vi "Teleop.vi"(10 "Match Info":T1={"Autonomous Elapsed Seconds"=0.0, "TeleOp Elapsed Seconds"=0.0, "Disabled Elapsed Seconds"=0.0, "Visited Autonomous"=FALSE, "Visited TeleOp"=FALSE, "Visited Disabled"=FALSE, "Autonomous Settings"={"Autonomous Style"=enum."Independent", "VI Refnum"=refnum}}, 11 "Call Context":T2) -> ()   [LabVIEW 2011]
doc: "This VI is called for each TeleOp packet received from the DS where the robot is not disabled. It is often used to read from the joysticks and update I/O or to update setpoints for timed control loops. It should complete and return within 20 milliseconds or it may miss DS packets."
uses:
  <vilib>/Rock Robotics/WPI/DriverStation/WPI_DriverStationDerivedRobotMode.ctl
  <vilib>/Rock Robotics/WPI/DriverStation/WPI_DriverStationMatch Info.ctl
  <vilib>/Rock Robotics/WPI/Relay/WPI_RelayValue.ctl
  Robot Global Data.vi
  <vilib>/Rock Robotics/WPI/RobotDrive/WPI_RobotDriveArcadeDrive_Standard(NoSaturation).vi
  <vilib>/Rock Robotics/WPI/Compressor/WPI_CompressorGetSetRefNum.vi
panel:
  in  "Time (msec)":u32=500
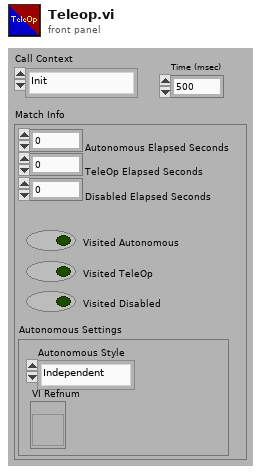
[diagram p1: front panel]
types:
  T1 = typedef "WPI_DriverStationMatch Info.ctl" = cluster{"Autonomous Elapsed Seconds":dbl, "TeleOp Elapsed Seconds":dbl, "Disabled Elapsed Seconds":dbl, "Visited Autonomous":bool, "Visited TeleOp":bool, "Visited Disabled":bool, "Autonomous Settings":cluster{"Autonomous Style":enum16{"Iterative", "Independent"}, "VI Refnum":refnum<vi>}}
  T2 = typedef "WPI_DriverStationDerivedRobotMode.ctl" = enum16{"Init", "Execute", "Stop"}
  T3 = typedef "WPI_RobotDriveDevRef.ctl" = cluster{"DevStatus":errorcluster, "Motors[]":T4[], "Square Inputs":bool, "Max Output":dbl, "Isochronous":bool}
  T4 = typedef "WPI_MotorControlDeviceRef.ctl" = cluster{"DeviceStatus":errorcluster, "Type":enum16{"PWM", "CAN"}, "PWM":cluster{"Digital Module":T5, "PWM Channel":T6, "DeadBand":T7}, "CAN":cluster{"Device Number":u8, "Control Mode":T8, "Semaphore":T9, "Max Vout":dbl}, "Invert":bool, "TransformRef":T10, "InvTransformRef":T10}
  T5 = typedef "FPGA_TypedefDigitalModule.ctl" = enum16{"Digital Module 1", "Digital Module 2"}
  T6 = typedef "FPGA_DIOPWMChannel.ctl" = enum8{"PWM 1", "PWM 2", "PWM 3", "PWM 4", "PWM 5", "PWM 6", "PWM 7", "PWM 8", "PWM 9", "PWM 10", "Invalid"}
  T7 = typedef "WPI_PWMDeadband.ctl" = cluster{"Name":string, "maxPositivePwm":i32, "minPositivePwm":i32, "centerPwm":i32, "maxNegativePwm":i32, "minNegativePwm":i32, "angularRange":u16}
  T8 = typedef "WPI_CANJaguar_ControlMode.ctl" = enum8{"Percent VBus", "Current", "Speed", "Position", "Voltage"}
  T9 = typedef "Semaphore RefNum" = refnum<k1>
  T10 = typedef "WPI_PWMTransform_ConPane.ctl" = refnum<vi>
  T11 = typedef "WPI_JoystickDevRef.ctl" = cluster{"Device":T12}
  T12 = typedef "WPI_JoystickDeviceEnum.ctl" = enum16{"USB 1", "USB 2", "USB 3", "USB 4", "Kinect 1", "Kinect 2"}
  T13 = typedef "WPI_JoystickButtonState.ctl" = cluster{"Button 1":bool, "Button 2":bool, "Button 3":bool, "Button 4":bool, "Button 5":bool, "Button 6":bool, "Button 7":bool, "Button 8":bool, "Button 9":bool, "Button 10":bool, "Button 11":bool, "Button 12":bool}
  T14 = cluster{"axis 1 (x)":dbl, "axis 2 (y)":dbl, "axis 3 (throttle)":dbl, "axis 4":dbl, "axis 5":dbl, "axis 6":dbl}
  T15 = typedef "WPI_RelayDevRef.ctl" = cluster{"DevStatus":errorcluster, "Relay Channel":T16, "Digital Module":T5, "Relay Direction":T17}
  T16 = typedef "FPGA_DIORelayChannel.ctl" = enum8{"Relay 1", "Relay 2", "Relay 3", "Relay 4", "Relay 5", "Relay 6", "Relay 7", "Relay 8", "Invalid"}
  T17 = typedef "WPI_RelayDirection.ctl" = enum16{"Both directions", "Forward only", "Reverse only"}
  T18 = typedef "WPI_CompressorDevRef.ctl" = cluster{"DevStatus":errorcluster, "DigitalInputDevRef":T19, "RelayDevRef":T15}
  T19 = typedef "WPI_DigitalInputDevRef.ctl" = cluster{"DevStatus":errorcluster, "DIO Channel":T20, "Digital Module":T5}
  T20 = typedef "FPGA_DIOChannel.ctl" = enum8{"DIO 1", "DIO 2", "DIO 3", "DIO 4", "DIO 5", "DIO 6", "DIO 7", "DIO 8", "DIO 9", "DIO 10", "DIO 11", "DIO 12", "DIO 13", "DIO 14", "Invalid"}
  T21 = typedef "WPI_RelayValue.ctl" = enum16{"Off", "On", "Forward", "Reverse"}
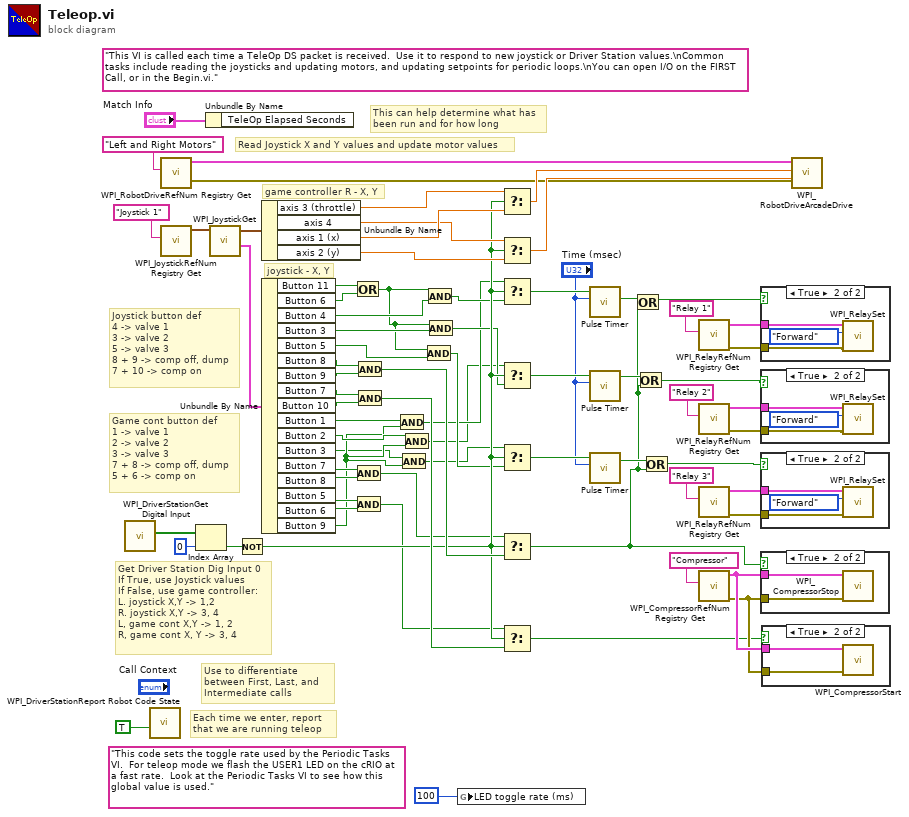
[diagram p0: block diagram]
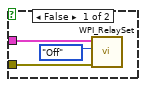
[diagram p2: hidden frame]
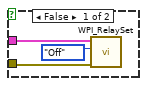
[diagram p3: hidden frame]
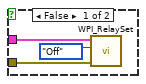
[diagram p4: hidden frame]
diagram:
  (unwired) "This code sets the toggle rate used by the Periodic Tasks VI.  For teleop mode we flash the USER1 LED on the cRIO at a fast rate.  Look at the Periodic Tasks VI to see how this global value is used."
  (unwired) "This VI is called each time a TeleOp DS packet is received.  Use it to respond to new joystick or Driver Station values.\nCommon tasks include reading the joysticks and updating motors, and updating setpoints for periodic loops.\nYou can open I/O on the FIRST Call, or in the Begin.vi."
  # "Joystick button def\n4 -> valve 1\n3 -> valve 2\n5 -> valve 3\n8 + 9 -> comp off, dump\n7 + 10 -> comp on"
  # "joystick - X, Y"
  # "game controller R - X, Y"
  # "Game cont button def\n1 -> valve 1\n2 -> valve 2\n3 -> valve 3\n7 + 8 -> comp off, dump\n5 + 6 -> comp on"
  # "Get Driver Station Dig Input 0\nIf True, use Joystick values\nIf False, use game controller:\nL. joystick X,Y -> 1,2\nR. joystick X,Y -> 3, 4\nL, game cont X,Y -> 1, 2\nR, game cont X, Y -> 3, 4"
  # "Each time we enter, report that we are running teleop"
  # "Use to differentiate between First, Last, and Intermediate calls"
  # "This can help determine what has\nbeen run and for how long"
  # "Read Joystick X and Y values and update motor values"
  n1 = call <vilib>:"WPI_DriverStationGet Digital Input.vi"() -> ("Driver Station Digital Input (1-8)"=w60:bool[])  [unwired: 11 in]
  n2 = call <vilib>:"WPI_DriverStationReport Robot Code State.vi"("TeleOp"=TRUE ("Autonomous")) -> ()  [unwired: 10 in, 1 out]
  n3 = call <vilib>:"WPI_RobotDriveRefNum Registry Get.vi"("refnum name"="Left and Right Motors") -> ("error out"=w24:errorcluster, "RobotDriveDevRef"=w65:T3)  [unwired: 1 in, 8 out]
  n4 = call <vilib>:"WPI_JoystickRefNum Registry Get.vi"("refnum name"="Joystick 1") -> ("JoystickDevRef"=w68:T11)  [unwired: 1 in, 9 out]
  n5 = Index Array(array=w60, index=0) -> (element=w52:bool)
  n6 = Unbundle By Name("Match Info") -> ()  [unwired: 1 out]
  n7 = call <vilib>:"WPI_JoystickGet.vi"("JoystickDevRef"=w68) -> ("Buttons"=w61:T13, "Axes"=w70:T14)  [unwired: 1 in, 4 out]
  n8 = Not(x=w52) -> (.not. x?=w33:bool)
  n9 = Unbundle By Name(w70) -> ("axis 3 (throttle)"=w54:dbl, "axis 4"=w53:dbl, "axis 1 (x)"=w55:dbl, "axis 2 (y)"=w56:dbl)
  n10 = Unbundle By Name(w61) -> ("Button 11"=w16:bool, "Button 6"=w15:bool, "Button 4"=w14:bool, "Button 3"=w12:bool, "Button 5"=w9:bool, "Button 8"=w51:bool, "Button 9"=w50:bool, "Button 7"=w46:bool, "Button 10"=w45:bool, "Button 1"=w7:bool, "Button 2"=w5:bool, "Button 3"=w2:bool, "Button 7"=w30:bool, "Button 8"=w28:bool, "Button 5"=w27:bool, "Button 6"=w26:bool, "Button 9"=w4:bool)
  n11 = Or(x=w16, y=w15) -> (x .or. y?=w10:bool)
  n12 = And(x=w30, y=w28) -> (x .and. y?=w31:bool)
  n13 = And(x=w27, y=w26) -> (x .and. y?=w29:bool)
  n14 = And(x=w51, y=w50) -> (x .and. y?=w35:bool)
  n15 = And(x=w46, y=w45) -> (x .and. y?=w34:bool)
  n16 = And(x=w7, y=w4) -> (x .and. y?=w6:bool)
  n17 = And(x=w2, y=w4) -> (x .and. y?=w1:bool)
  n18 = And(x=w5, y=w4) -> (x .and. y?=w3:bool)
  n19 = And(x=w10, y=w9) -> (x .and. y?=w8:bool)
  n20 = And(x=w10, y=w14) -> (x .and. y?=w13:bool)
  n21 = And(x=w10, y=w12) -> (x .and. y?=w11:bool)
  n22 = global write "Robot Global Data.vi" "LED toggle rate (ms)"(u32 100 ("LED ms toggle rate")) -> ()
  n23 = Select(t=w54, s=w33, f=w55) -> (s? t:f=w58:dbl)
  n24 = Select(t=w53, s=w33, f=w56) -> (s? t:f=w57:dbl)
  n25 = Select(t=w6, s=w33, f=w13) -> (s? t:f=w38:bool)
  n26 = Select(t=w3, s=w33, f=w11) -> (s? t:f=w37:bool)
  n27 = Select(t=w1, s=w33, f=w8) -> (s? t:f=w36:bool)
  n28 = Select(t=w31, s=w33, f=w35) -> (s? t:f=w17:bool)
  n29 = Select(t=w29, s=w33, f=w34) -> (s? t:f=w32:bool)
  n30 = call "Pulse Timer.vi"("Time"="Time (msec)", "Start"=w38) -> ("Timeout"=w23:bool)  [unwired: 8 in, 1 out]
  n31 = call "Pulse Timer.vi"("Time"="Time (msec)", "Start"=w37) -> ("Timeout"=w20:bool)  [unwired: 8 in, 1 out]
  n32 = call "Pulse Timer.vi"("Time"="Time (msec)", "Start"=w36) -> ("Timeout"=w22:bool)  [unwired: 8 in, 1 out]
  n33 = Or(x=w23, y=w17) -> (x .or. y?=w18:bool)
  n34 = Or(x=w20, y=w17) -> (x .or. y?=w19:bool)
  n35 = Or(x=w22, y=w17) -> (x .or. y?=w21:bool)
  n36 = call <vilib>:"WPI_RelayRefNum Registry Get.vi"("refnum name"="Relay 1") -> ("error out"=w41:errorcluster, "RelayDevRef"=w43:T15)  [unwired: 9 in]
  n37 = call <vilib>:"WPI_RelayRefNum Registry Get.vi"("refnum name"="Relay 2") -> ("error out"=w40:errorcluster, "RelayDevRef"=w42:T15)  [unwired: 9 in]
  n38 = call <vilib>:"WPI_RelayRefNum Registry Get.vi"("refnum name"="Relay 3") -> ("error out"=w39:errorcluster, "RelayDevRef"=w44:T15)  [unwired: 9 in]
  n39 = call <vilib>:"WPI_CompressorRefNum Registry Get.vi"("refnum name"="Compressor") -> ("error out"=w47:errorcluster, "CompressorDevRef"=w48:T18)  [unwired: 9 in]
  n40 = case shown="True" w18 {
    tunnel: w43 -> [w74 w77]
    tunnel: w41 -> [w73 w76]
    frame False {
      n41 = call <vilib>:"WPI_RelaySet.vi"("error in (no error)"=w73, "RelayValue"=WPI_RelayValue."Off", "RelayDevRef"=w74) -> ()  [unwired: 7 in, 2 out]
    }
    frame True {
      n42 = call <vilib>:"WPI_RelaySet.vi"("error in (no error)"=w76, "RelayValue"=WPI_RelayValue."Forward", "RelayDevRef"=w77) -> ()  [unwired: 7 in, 2 out]
    }
  }
  n43 = case shown="True" w19 {
    tunnel: w42 -> [w80 w83]
    tunnel: w40 -> [w79 w82]
    frame False {
      n44 = call <vilib>:"WPI_RelaySet.vi"("error in (no error)"=w79, "RelayValue"=WPI_RelayValue."Off", "RelayDevRef"=w80) -> ()  [unwired: 7 in, 2 out]
    }
    frame True {
      n45 = call <vilib>:"WPI_RelaySet.vi"("error in (no error)"=w82, "RelayValue"=WPI_RelayValue."Forward", "RelayDevRef"=w83) -> ()  [unwired: 7 in, 2 out]
    }
  }
  n46 = case shown="True" w21 {
    tunnel: w44 -> [w86 w89]
    tunnel: w39 -> [w85 w88]
    frame False {
      n47 = call <vilib>:"WPI_RelaySet.vi"("error in (no error)"=w85, "RelayValue"=WPI_RelayValue."Off", "RelayDevRef"=w86) -> ()  [unwired: 7 in, 2 out]
    }
    frame True {
      n48 = call <vilib>:"WPI_RelaySet.vi"("error in (no error)"=w88, "RelayValue"=WPI_RelayValue."Forward", "RelayDevRef"=w89) -> ()  [unwired: 7 in, 2 out]
    }
  }
  n49 = case shown="True" w17 {
    tunnel: w48 -> [_ w92]
    tunnel: w47 -> [_ w91]
    frame False {
    }
    frame True {
      n50 = call <vilib>:"WPI_CompressorStop.vi"("error in (no error)"=w91, "CompressorDevRef"=w92) -> ()  [unwired: 8 in, 2 out]
    }
  }
  n51 = case shown="True" w32 {
    tunnel: w48 -> [_ w94]
    tunnel: w47 -> [_ w93]
    frame False {
    }
    frame True {
      n52 = call <vilib>:"WPI_CompressorStart.vi"("error in (no error)"=w93, "CompressorDevRef"=w94) -> ()  [unwired: 8 in, 2 out]
    }
  }
  n53 = call-poly <vilib>:"WPI_RobotDriveArcadeDrive.vi"("error in (no error)"=w24, "Y axis value"=w57, "X axis value"=w58, "RobotDriveDevRef"=w65) -> ()  [unwired: 6 in, 2 out]
